vi "Normalize Connect Flags.vi"(9 "Payload":T1, 11 "Connect Flags in":T2) -> (1 "Payload out":T1, 3 "Connect Flags out":T2)   [LabVIEW 2013, in "CONNECT.lvclass"]
uses:
  CONNECT.lvclass
  ConnectFlags -- cluster.ctl
  ConnectPayload -- cluster.ctl
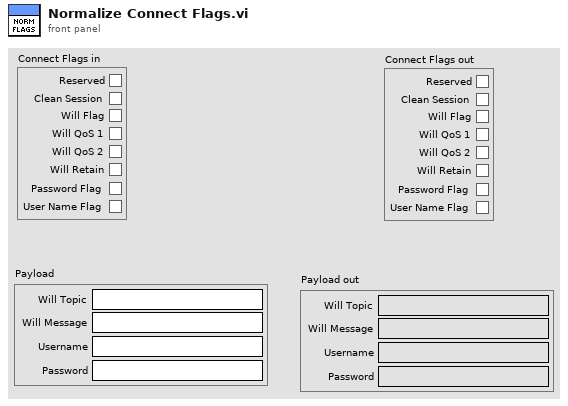
[diagram p1: front panel]
types:
  T1 = typedef "CONNECT.lvclass/ConnectPayload -- cluster.ctl" = cluster{"Will Topic":string, "Will Message":string, "Username":string, "Password":string}
  T2 = typedef "CONNECT.lvclass/ConnectFlags -- cluster.ctl" = cluster{"Reserved":bool, "Clean Session":bool, "Will Flag":bool, "Will QoS 1":bool, "Will QoS 2":bool, "Will Retain":bool, "Password Flag":bool, "User Name Flag":bool}
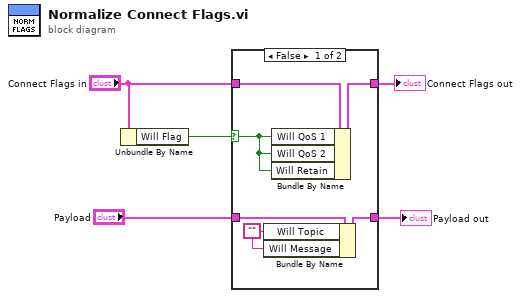
[diagram p0: block diagram]
diagram:
  n1 = Unbundle By Name("Connect Flags in") -> ("Will Flag"=w3:bool)
  n2 = case shown="False" w3 {
    selector: w3 -> [w9 _]
    tunnel: [w11 w13] -> w5
    tunnel: "Connect Flags in" -> [w10 w13]
    tunnel: "Payload" -> [w8 w12]
    tunnel: [w7 w12] -> w1
    frame False {
      w6 = ""
      n3 = Bundle By Name(cluster=w8, "Will Topic"=w6, "Will Message"=w6) -> (w7:T1)
      n4 = Bundle By Name(cluster=w10, "Will QoS 1"=w9, "Will QoS 2"=w9, "Will Retain"=w9) -> (w11:T2)
    }
    frame True {
    }
  }
  "Connect Flags out" <- w5
  "Payload out" <- w1
